vi "Get Controls Data.vi"(8 "error in (no error)":errorcluster, 11 "VI in":refnum<class "VI.lvclass">) -> (0 "error out":errorcluster, 3 "VI out":refnum<class "VI.lvclass">)   [LabVIEW 2020, in "VI Properties Editor.lvlib" / "VI.lvclass"]
doc: "Gets all controls data for <B>VI in</B>."
uses:
  VI.lvclass
  Control/Control.lvclass
  VI Properties Editor.lvlib
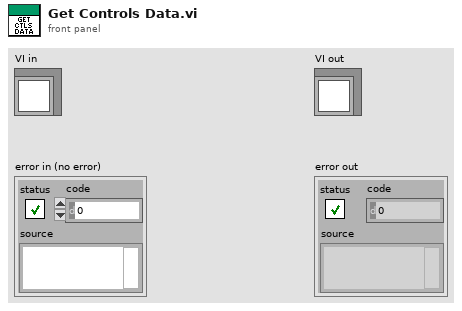
[diagram p1: front panel]
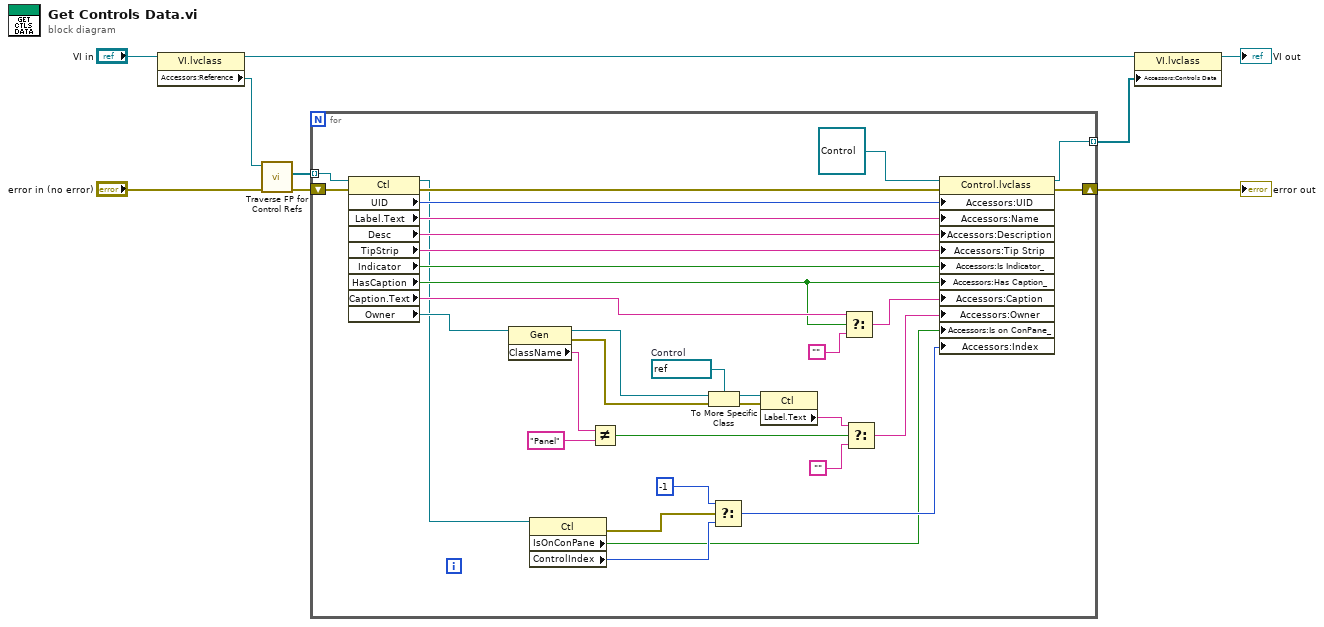
[diagram p0: block diagram]
diagram:
  n1 = property class="VI.lvclass"(reference="VI in") -> (reference out=w7:refnum<class "VI.lvclass">, "Accessors:Reference"=w3:refnum<vi>)  [unwired: 1 in, 1 out]
  n2 = call "Traverse FP for Control Refs.vi"("error in (no error)"="error in (no error)", "VI Ref"=w3) -> ("error out"=w2:errorcluster, "Control Refs"=w1:refnum<vi>[])  [unwired: 7 in, 1 out]
  n3 = for {
    shift-right: [w10] -> w9
    shift-left: w2 -> [w32]
    tunnel: [w40] -> w6 mode=indexing
    tunnel: w1 -> [w33] mode=indexing
    w28 = refnum<vi> refnum  # Control
    n4 = property class="Ctl"(reference=w33, error in=w32) -> (reference out=w16:refnum<vi>, error out=w41:errorcluster, "UID"=w39:i32, "Label.Text"=w38:string, "Desc"=w37:string, "TipStrip"=w36:string, "Indicator"=w35:bool, "HasCaption"=w19:bool, "Caption.Text"=w20:string, "Owner"=w31:refnum<vi>)
    n5 = property class="Gen"(reference=w31) -> (reference out=w26:refnum<vi>, error out=w27:errorcluster, "ClassName"=w30:string)  [unwired: 1 in]
    n6 = property class="Ctl"(reference=w16) -> (error out=w15:errorcluster, "IsOnConPane"=w11:bool, "ControlIndex"=w12:i32)  [unwired: 1 in, 1 out]
    n7 = Not Equal?(x=w30, y="Panel") -> (x != y?=w24:bool)
    n8 = To More Specific Class(target class=w28, reference=w26, error in=w27) -> (specific class reference=w25:refnum<vi>, error out=w21:errorcluster)
    n9 = Select(t=-1, s=w15, f=w12) -> (s? t:f=w13:i32)
    n10 = property class="Ctl"(reference=w25, error in=w21) -> ("Label.Text"=w22:string)  [unwired: 2 out]
    n11 = Select(t=w20, s=w19, f="") -> (s? t:f=w17:string)
    n12 = Select(t=w22, s=w24, f="") -> (s? t:f=w34:string)
    n13 = property class="Control.lvclass"(reference=refnum<class "Control.lvclass"> refnum ("Control"), error in=w41, "Accessors:UID"=w39, "Accessors:Name"=w38, "Accessors:Description"=w37, "Accessors:Tip Strip"=w36, "Accessors:Is Indicator_"=w35, "Accessors:Has Caption_"=w19, "Accessors:Caption"=w17, "Accessors:Owner"=w34, "Accessors:Is on ConPane_"=w11, "Accessors:Index"=w13) -> (reference out=w40:refnum<class "Control.lvclass">, error out=w10:errorcluster)
  }
  "error out" <- w9
  n14 = property class="VI.lvclass"(reference=w7, "Accessors:Controls Data"=w6) -> (reference out=→"VI out":refnum<class "VI.lvclass">)  [unwired: 1 in, 1 out]
